vi "Read DC meter.vi"(7 "abort reference":refnum<vi>, 8 "error in (no error)":errorcluster, 11 "DC meter":T1={"DC meter type"=enum."H/A/K 3458", "DC meter VISA"="", "NPLC"=10, "No of readings"=3, "status ref"=refnum}) -> (0 "error out":errorcluster, 2 "DC readings":dbl[](array[numeric]), 3 "DC meter out":T1={"DC meter type"=enum."H/A/K 3458", "DC meter VISA"="", "NPLC"=10, "No of readings"=3, "status ref"=refnum})   [LabVIEW 2020]
uses:
  Type definitions/DC meter.ctl
  Type definitions/DC meter type.ctl
  <vilib>/Utility/error.llb/Error Cluster From Error Code.vi
  external libraries/3458A Basic Driver/Public/Data/Read Measurement(Single Point).vi
  <vilib>/ErrorRing/Error Ring.xnode
  external libraries/Fluke 8508/Fluke 8508.lvlib
  external libraries/3458A Basic Driver/3458A Basic Driver.lvlib
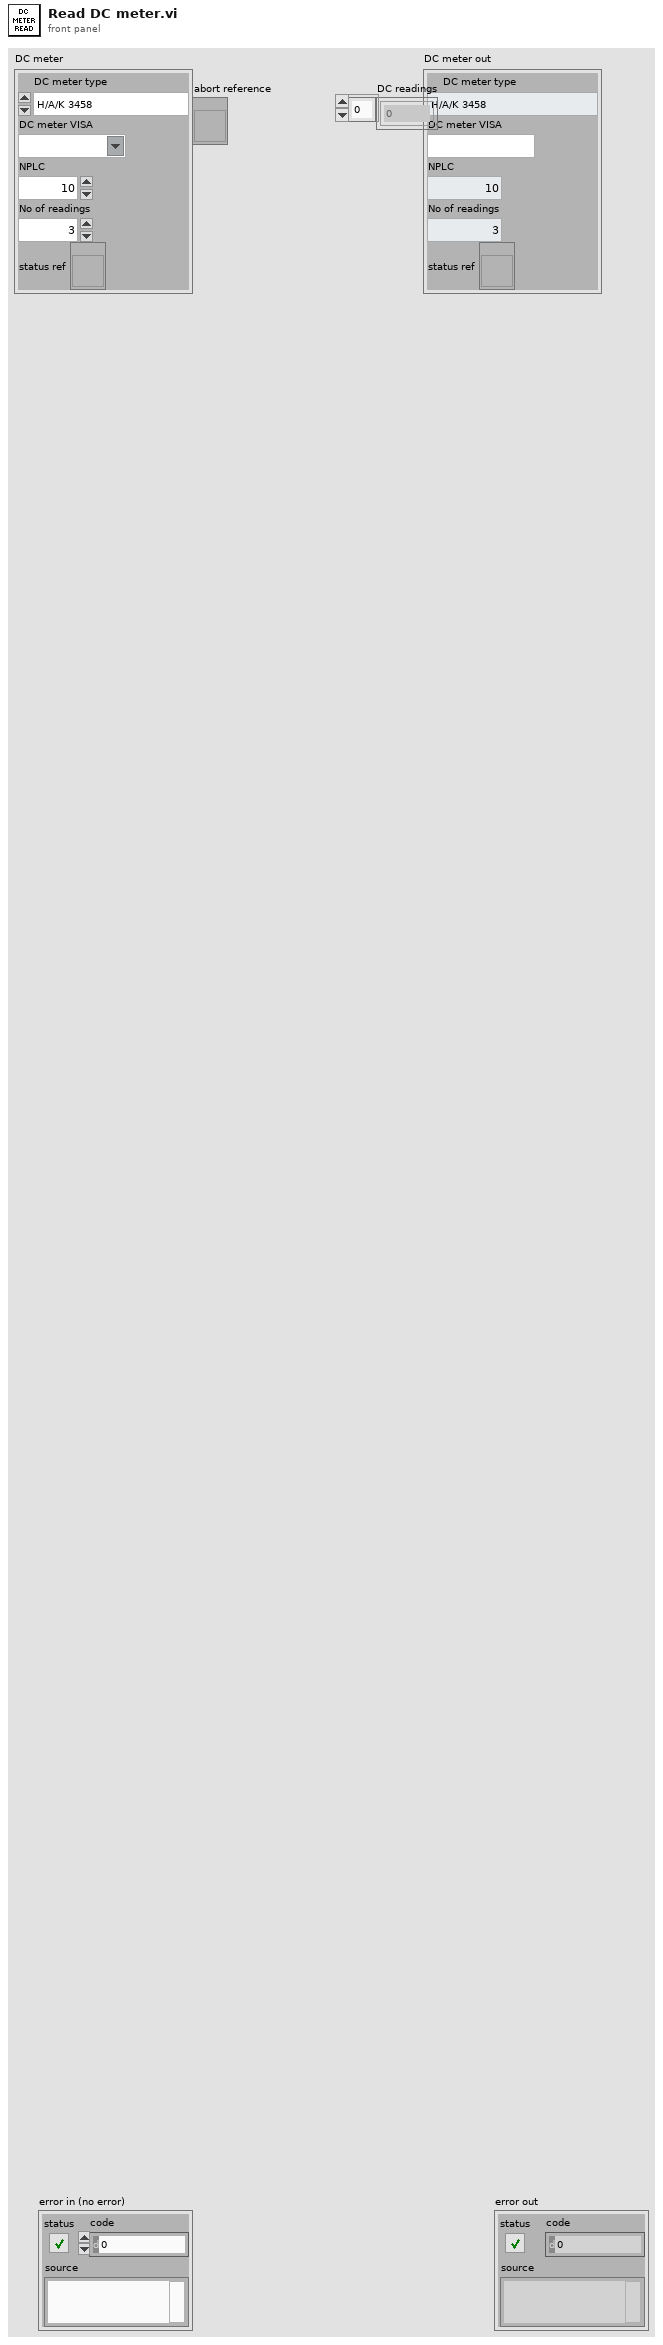
[diagram p1: front panel]
types:
  T1 = typedef "DC meter.ctl" = cluster{"DC meter type":T2, "DC meter VISA":refnum<visa-resource-name>, "NPLC":i32, "No of readings":i32, "status ref":refnum<vi>}
  T2 = typedef "DC meter type.ctl" = enum16{"H/A/K 3458", "FLuke 8508A", "dummy"}
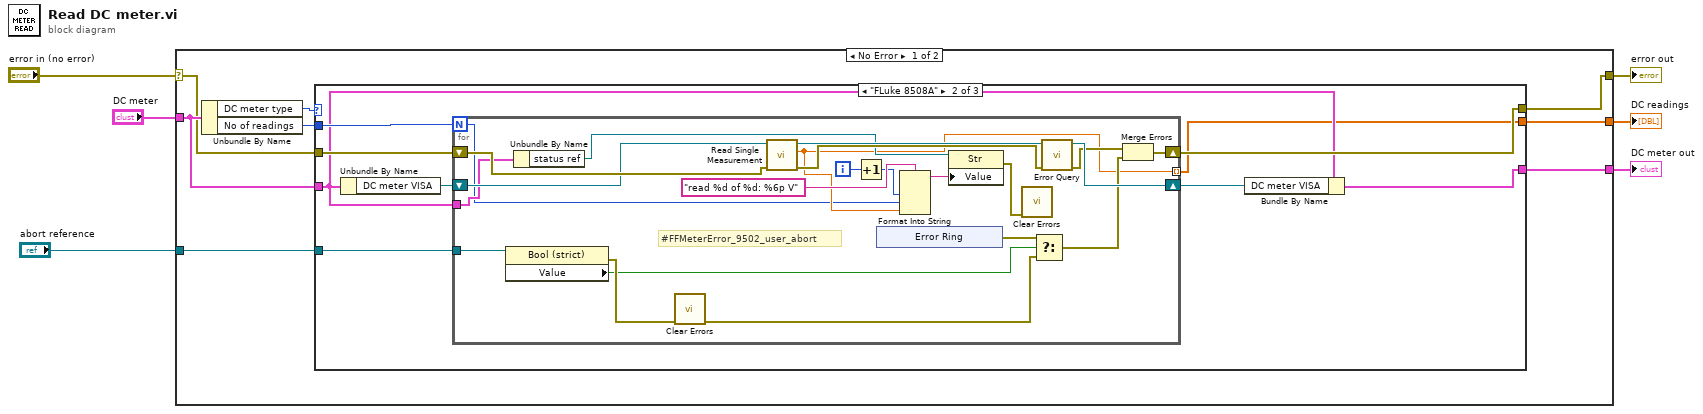
[diagram p0: block diagram]
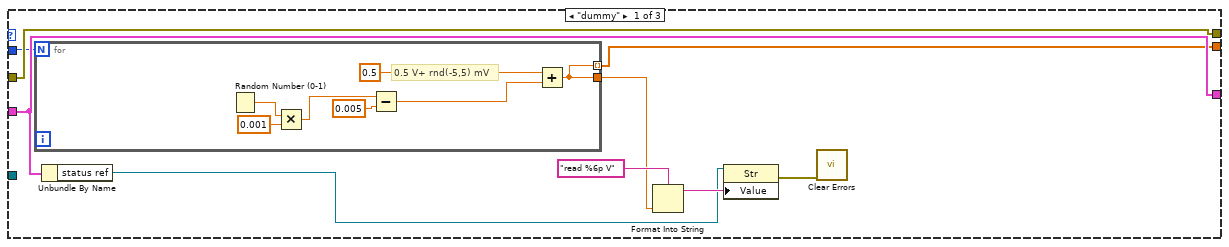
[diagram p2: hidden frame]
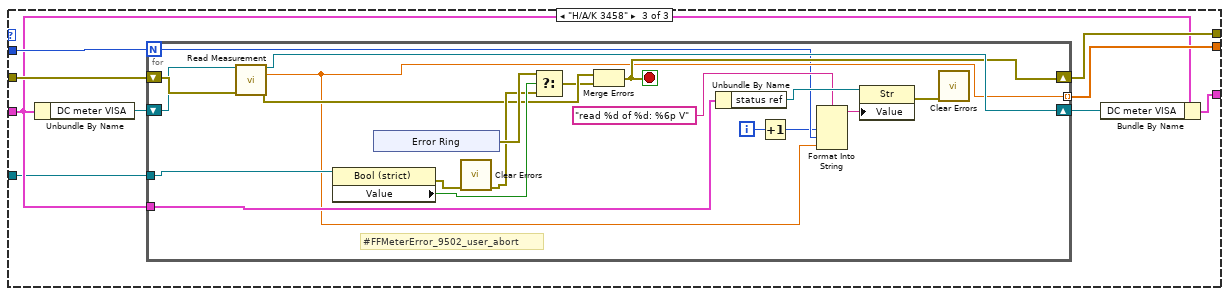
[diagram p3: hidden frame]
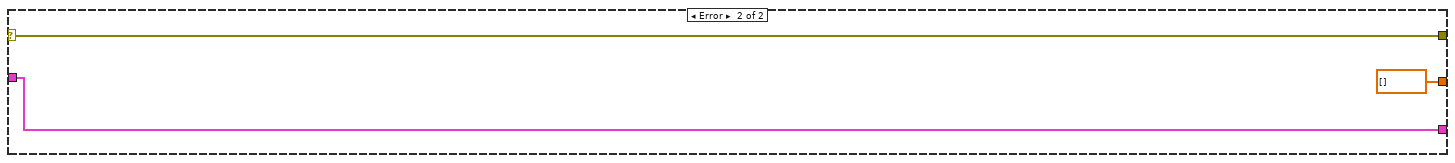
[diagram p4: hidden frame]
diagram:
  n1 = case shown="No Error" "error in (no error)" {
    selector: "error in (no error)" -> [w10 w103]
    tunnel: [w14 w103] -> w6
    tunnel: "DC meter" -> [w12 w102]
    tunnel: [w8 w102] -> w4
    tunnel: [w11 dbl[] [] ("Measurements")] -> w3
    tunnel: "abort reference" -> [w7 _]
    frame No Error {
      n2 = Unbundle By Name(w12) -> ("DC meter type"=w13:T2, "No of readings"=w9:i32)
      n3 = case shown="\"FLuke 8508A\"" w13 {
        tunnel: w10 -> [w23 w39 w75]
        tunnel: [w23 w36 w74] -> w14
        tunnel: w12 -> [w19 w33 w69]
        tunnel: [w19 w37 w68] -> w8
        tunnel: [w16 w32 w72] -> w11
        tunnel: w9 -> [w17 w34 w71]
        tunnel: w7 -> [_ w31 w67]
        frame "dummy" {
          n4 = for {
            N: w17 -> [_]
            tunnel: [w24] -> w16 mode=indexing
            tunnel: [w24] -> w15
            # "0.5 V+ rnd(-5,5) mV"
            n5 = Random Number (0-1)() -> (number: 0 to 1=w30:dbl)
            n6 = Multiply(x=w30, y=0.001) -> (x*y=w28:dbl)
            n7 = Subtract(x=w28, y=0.005) -> (x-y=w26:dbl)
            n8 = Add(x=0.5, y=w26) -> (x+y=w24:dbl)
          }
          n9 = Unbundle By Name(w19) -> ("status ref"=w18:refnum<vi>)
          n10 = Format Into String(format string="read %6p V", w15) -> (resulting string=w22:string)  [unwired: 2 in, 1 out]
          n11 = property class="Str"(reference=w18, "Value"=w22) -> (error out=w20:errorcluster)  [unwired: 1 in, 1 out]
          n12 = call <vilib>:"Clear Errors.vi"("error in (no error)"=w20) -> ()  [unwired: 5 in, 2 out]
        }
        frame "FLuke 8508A" {
          n13 = Unbundle By Name(w33) -> ("DC meter VISA"=w38:refnum<visa-resource-name>)
          n14 = for {
            N: w34 -> [w42]
            tunnel: [w43] -> w32 mode=indexing
            shift-right: [w44] -> w36
            shift-left: w39 -> [w61]
            shift-right: [w57] -> w35
            shift-left: w38 -> [w60]
            tunnel: w33 -> [w53]
            tunnel: w31 -> [w46]
            i -> [w41]
            # "#FFMeterError_9502_user_abort"
            n15 = property class="Bool (strict)"(reference=w46) -> (error out=w51:errorcluster, "Value"=w50:bool)  [unwired: 1 in, 1 out]
            n16 = Unbundle By Name(w53) -> ("status ref"=w56:refnum<vi>)
            n17 = call <vilib>:"Clear Errors.vi"("error in (no error)"=w51) -> ("error out"=w48:errorcluster)  [unwired: 5 in, 1 out]
            n18 = call "Read Single Measurement.vi"("error in (no error)"=w61, "VISA resource name"=w60) -> ("error out"=w59:errorcluster, "Measurement"=w43:dbl, "VISA resource name out"=w58:refnum<visa-resource-name>)  [unwired: 7 in]
            n19 = Increment(x=w41) -> (x+1=w40:i32)
            n20 = xnode "Error Ring"() -> ("error out"=w49:errorcluster)
            n21 = Format Into String(format string="read %d of %d: %6p V", w40, w42, w43) -> (resulting string=w52:string)  [unwired: 2 in, 1 out]
            n22 = property class="Str"(reference=w56, "Value"=w52) -> (error out=w55:errorcluster)  [unwired: 1 in, 1 out]
            n23 = call <vilib>:"Clear Errors.vi"("error in (no error)"=w55) -> ()  [unwired: 5 in, 2 out]
            n24 = Select(t=w49, s=w50, f=w48) -> (s? t:f=w47:errorcluster)
            n25 = call "Error Query.vi"("error in (no error)"=w59, "VISA resource name"=w58) -> ("error out"=w45:errorcluster, "VISA resource name out"=w57:refnum<visa-resource-name>)  [unwired: 6 in, 2 out]
            n26 = Merge Errors(w45, w47) -> (w44:errorcluster)
          }
          n27 = Bundle By Name(cluster=w33, "DC meter VISA"=w35) -> (w37:T1)
        }
        frame "H/A/K 3458" {
          n28 = Unbundle By Name(w69) -> ("DC meter VISA"=w73:refnum<visa-resource-name>)
          n29 = for {
            N: w71 -> [w78]
            tunnel: [w79] -> w72 mode=indexing
            shift-right: [w80] -> w74
            shift-left: w75 -> [w95]
            shift-right: [w89] -> w70
            shift-left: w73 -> [w94]
            tunnel: w69 -> [w88]
            tunnel: w67 -> [w83]
            i -> [w77]
            stop <- w80 stop-if-true
            # "#FFMeterError_9502_user_abort"
            n30 = call-poly "Read Measurement.vi"("VISA resource name"=w94, "error in (no error)"=w95) -> ("VISA resource name out"=w89:refnum<visa-resource-name>, "Measurement"=w79:dbl, "error out"=w82:errorcluster)  [unwired: 11 in]
            n31 = property class="Bool (strict)"(reference=w83) -> (error out=w87:errorcluster, "Value"=w86:bool)  [unwired: 1 in, 1 out]
            n32 = xnode "Error Ring"() -> ("error out"=w85:errorcluster)
            n33 = call <vilib>:"Clear Errors.vi"("error in (no error)"=w87) -> ("error out"=w84:errorcluster)  [unwired: 5 in, 1 out]
            n34 = Select(t=w85, s=w86, f=w84) -> (s? t:f=w81:errorcluster)
            n35 = Merge Errors(w82, w81) -> (w80:errorcluster)
            n36 = Unbundle By Name(w88) -> ("status ref"=w92:refnum<vi>)
            n37 = Increment(x=w77) -> (x+1=w76:i32)
            n38 = Format Into String(format string="read %d of %d: %6p V", w76, w78, w79) -> (resulting string=w93:string)  [unwired: 2 in, 1 out]
            n39 = property class="Str"(reference=w92, "Value"=w93) -> (error out=w91:errorcluster)  [unwired: 1 in, 1 out]
            n40 = call <vilib>:"Clear Errors.vi"("error in (no error)"=w91) -> ()  [unwired: 5 in, 2 out]
          }
          n41 = Bundle By Name(cluster=w69, "DC meter VISA"=w70) -> (w68:T1)
        }
      }
    }
    frame Error {
    }
  }
  "error out" <- w6
  "DC meter out" <- w4
  "DC readings" <- w3
